vi "Pane Bounds to Panel Bounds.vi"(1 "Pane Bounds In":cluster{"Width":u32, "Height":u32}) -> (0 "Panel Bound Out":cluster{i32, i32, u32, u32})   [LabVIEW 2009, in "UI Panels.lvlib" / "Panels_XControl.xctl"]
uses:
  Panels_XControl.xctl
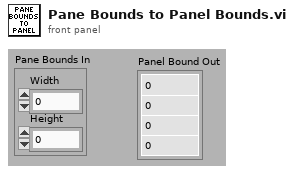
[diagram p1: front panel]
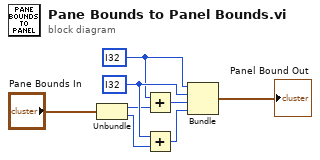
[diagram p0: block diagram]
diagram:
  w5 = i32 ?
  w4 = i32 ?
  n1 = Unbundle("Pane Bounds In") -> ("Width"=w2:u32, "Height"=w3:u32)
  n2 = Add(x=w4, y=w2) -> (x+y=w6:u32)
  n3 = Add(x=w5, y=w3) -> (x+y=w7:u32)
  n4 = Bundle(w4, w5, w6, w7) -> (→"Panel Bound Out":cluster{i32, i32, u32, u32})  [unwired: 1 in]
